vi "_information.vi"(10 "error in (no error)":errorcluster, 11 "MDPtr DVR":refnum<data-value>) -> (1 "Common":T1, 2 "error out":errorcluster, 3 "MDPtr DVR(dup)":refnum<data-value>)   [LabVIEW 2017, in "MDPtr.lvlib"]
uses:
  MDPtr.lvlib
  MDPtr TypeDef/MDPtr DataFrame-Memory.ctl
  MDPtr TypeDef/MDPtr DataFrame-Common.ctl
  <vilib>/Utility/Data Type/Type Definitions/Data Type.ctl
  _MDPtr Build Error Cluster.vi
  <vilib>/Utility/Data Type/NI_Data Type.lvlib
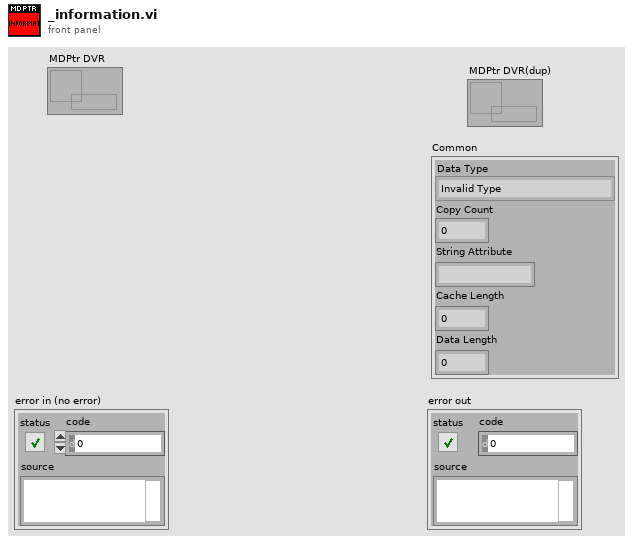
[diagram p1: front panel]
types:
  T1 = typedef "MDPtr.lvlib/MDPtr DataFrame-Common.ctl" = cluster{"Data Type":T2, "Copy Count":i32, "String Attribute":string, "Cache Length":i32, "Data Length":i32}
  T2 = typedef "NI_Data Type.lvlib/Data Type.ctl" = enum8{"Invalid Type", "Void", "I8", "I16", "I32", "I64", "U8", "U16", "U32", "U64", "Single Float", "Double Float", "Extended Float", "Single Complex", "Double Complex", "Extended Complex", "Enum U8", "Enum U16", "Enum U32", "Enum U64", "Single Float With Unit", "Double Float With Unit", "Extended Float With Unit", "Single Complex with Unit", "Double Complex with Unit", "Extended Complex with Unit", "Boolean", "String", "Path", "Picture", "Tag", "Array", "Cluster", "Variant", "LV Variant", "Waveform", "Timestamp", "Digital Waveform", "Digital Data", "ExpressData", "Refnum", "External Data", "VI", "Poly VI", "LabVIEW Class Instance", "Fixed Point"}
  T3 = typedef "MDPtr.lvlib/MDPtr DataFrame-Memory.ctl" = cluster{"Common":T1, "DVR":refnum<data-value>}
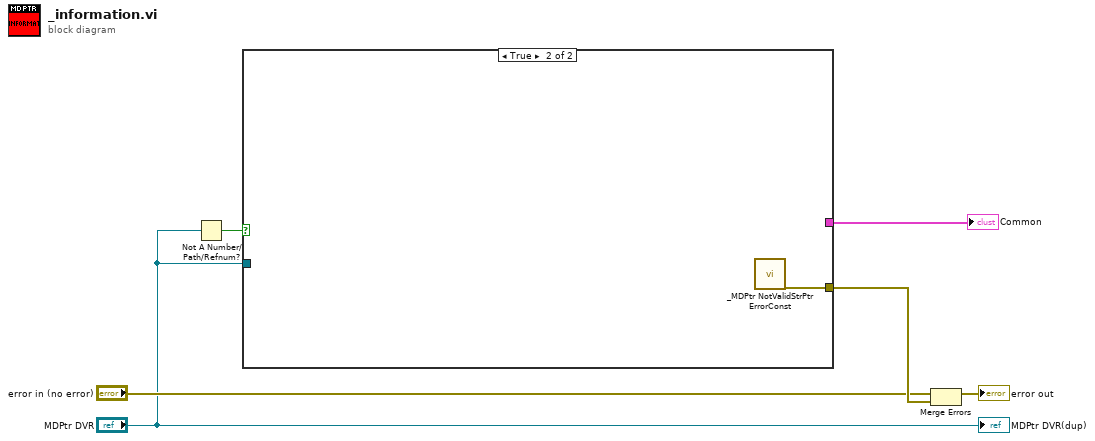
[diagram p0: block diagram]
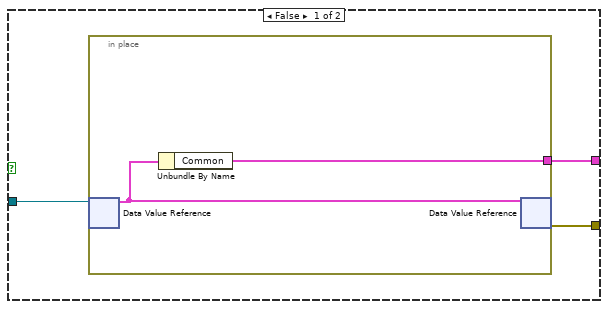
[diagram p2: hidden frame]
diagram:
  n1 = Not A Number/Path/Refnum?(number/path/refnum="MDPtr DVR") -> (NaN/Path/Refnum?=w2:bool)
  n2 = case shown="True" w2 {
    tunnel: [w9 w12] -> w6
    tunnel: "MDPtr DVR" -> [w8 _]
    tunnel: [w7 _] -> w1
    frame False {
      n3 = in-place {
        in-place-border: [w10] -> w7
        n4 = in-place-dvr #1(w8) -> (w11:T3)  [unwired: 1 out]
        n5 = Unbundle By Name(w11) -> ("Common"=w10:T1)
        n6 = in-place-dvr #1(w11) -> (w9:errorcluster)  [unwired: 1 out]
      }
    }
    frame True {
      n7 = call "_MDPtr NotValidStrPtr ErrorConst.vi"() -> ("error out"=w12:errorcluster)  [unwired: 19 in]
    }
  }
  "Common" <- w1
  n8 = Merge Errors("error in (no error)", w6) -> (→"error out":errorcluster)
  "MDPtr DVR(dup)" <- "MDPtr DVR"
